vi "CRDS Server.vi"(10 "nCRD in":refnum<class "nCRD.lvclass">, 11 "DVR In":refnum<data-value>) -> (3 "nCRD out":refnum<class "nCRD.lvclass">)   [LabVIEW 2016]
uses:
  <vilib>/MSR Consulting, LLC/General Reuse/Instrument/Instrument.lvclass
  <vilib>/MSR Consulting, LLC/General Reuse/Instrument/state.ctl
  CRD/nCRD.lvclass
  <vilib>/MSR Consulting, LLC/General Reuse/Session APIs/Session Log/System Log.lvclass
  <vilib>/MSR Consulting, LLC/General Reuse/Session APIs/_Session Fwk/Session - Root.lvclass
  <vilib>/MSR Consulting, LLC/General Reuse/Session APIs/File Access/Config Data/Config Data.lvclass
  C:/Program Files (x86)/National Instruments/LabVIEW 2016/vi.lib/MSR Consulting, LLC/General Reuse/CRDS/Main/CRDS.lvclass
  C:/Program Files (x86)/National Instruments/LabVIEW 2016/vi.lib/MSR Consulting, LLC/General Reuse/Instrument/Instrument.lvclass
  C:/Program Files (x86)/National Instruments/LabVIEW 2016/vi.lib/MSR Consulting, LLC/General Reuse/Session APIs/_Session Fwk/Session - Root.lvclass
  Data/Nicholas Data.lvclass
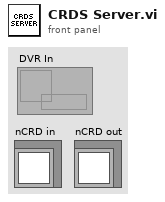
[diagram p1: front panel]
types:
  T1 = typedef "Instrument.lvclass/state.ctl" = enum8{"Configure", "Acquire", "Wait", "Quit", "Handle Error", "NOOP"}
  T2 = typedef "Session - Root.lvclass/Session Handle.ctl" = refnum<data-value>
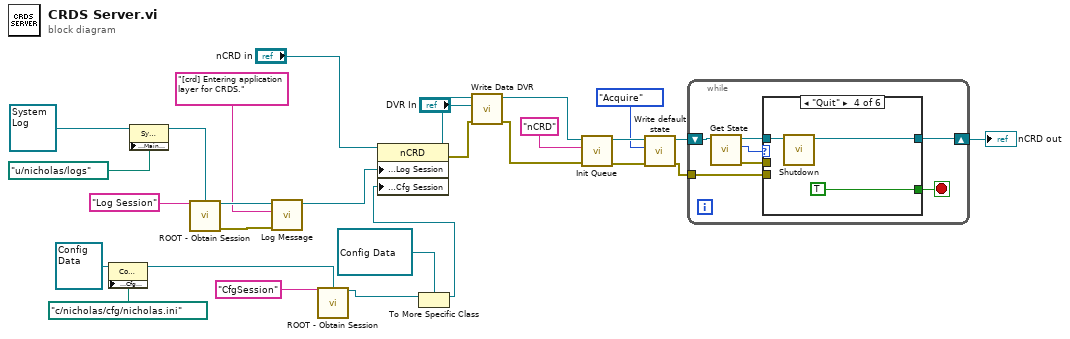
[diagram p0: block diagram]
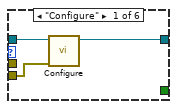
[diagram p2: hidden frame]
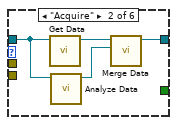
[diagram p3: hidden frame]
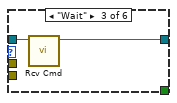
[diagram p4: hidden frame]
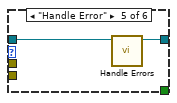
[diagram p5: hidden frame]
diagram:
  n1 = property class="Config Data"(reference=refnum<class "Config Data.lvclass"> refnum ("Config Data"), "Accessors:Cfg Path"=path "c:/nicholas/cfg/nicholas.ini" ("Cfg Path")) -> (reference out=w8:refnum<class "Config Data.lvclass">)  [unwired: 1 in, 1 out]
  n2 = property class="Sys Log"(reference=refnum<class "System Log.lvclass"> refnum ("Sys Log"), "Accessors:Main Path"=path "u:/nicholas/logs" ("Main Path")) -> (reference out=w16:refnum<class "System Log.lvclass">)  [unwired: 1 in, 1 out]
  n3 = call <vilib>:"ROOT - Obtain Session.vi"("Session Name ()"="Log Session", "OBJ - Session"=w16) -> ("Session Handle"=w13:T2, "error out"=w12:errorcluster)  [unwired: 11 in, 1 out]
  n4 = call <vilib>:"Log Message.vi"("error in"=w12, "MSG In"="[crd] Entering application layer for CRDS.", "session in"=w13) -> ("session out"=w10:T2)  [unwired: 7 in, 1 out]
  n5 = call <vilib>:"ROOT - Obtain Session.vi"("Session Name ()"="CfgSession", "OBJ - Session"=w8) -> ("Session Handle"=w3:T2)  [unwired: 11 in, 2 out]
  n6 = To More Specific Class(target class=refnum<data-value> refnum, reference=w3) -> (specific class reference=w1:refnum<data-value>)  [unwired: 1 in, 1 out]
  n7 = property class="nCRD"(reference="nCRD in", "Accessors:Log Session"=w10, "Accessors:Cfg Session"=w1) -> (reference out=w14:refnum<class "nCRD.lvclass">, error out=w5:errorcluster)  [unwired: 1 in]
  n8 = call "Write Data DVR.vi"("error in (no error)"=w5, "Data DVR"="DVR In", "nCRD in"=w14) -> ("error out"=w19:errorcluster, "nCRD out"=w28:refnum<class "nCRD.lvclass">)  [unwired: 7 in]
  n9 = call <vilib>:"Init Queue.vi"("error in"=w19, "queue_name"="nCRD", "Instrument in"=w28) -> ("error out"=w26:errorcluster, "Instrument out"=w25:refnum<class "nCRD.lvclass">)  [unwired: 7 in]
  n10 = call <vilib>:"Write default state.vi"("error in (no error)"=w26, "instr state"=state."Acquire", "Instrument in"=w25) -> ("error out"=w24:errorcluster, "Instrument out"=w23:refnum<class "nCRD.lvclass">)  [unwired: 7 in]
  n11 = while {
    shift-right: [w31] -> w20
    shift-left: w23 -> [w32]
    tunnel: w24 -> [w30]
    stop <- w34 stop-if-true
    n12 = call <vilib>:"Get State.vi"("Instrument in"=w32) -> ("error out"=w29:errorcluster, "default state"=w35:T1, "Instrument out"=w33:refnum<class "nCRD.lvclass">)  [unwired: 8 in]
    n13 = case shown="\"Quit\"" w35 {
      tunnel: [_ _ _ TRUE _ _] -> w34
      tunnel: w33 -> [w38 w42 w44 w46 w49 w50]
      tunnel: [w37 w41 w43 w45 w48 w50] -> w31
      tunnel: w30 -> [w36 _ _ _ _ _]
      tunnel: w29 -> [_ _ _ _ _ _]
      frame "Configure" {
        n14 = call-dynamic "Configure.vi"("error in"=w36, "nCRD in"=w38) -> ("nCRD out"=w37:refnum<class "nCRD.lvclass">)  [unwired: 8 in, 1 out]
      }
      frame "Acquire" {
        n15 = call-dynamic "Get Data.vi"("nCRD in"=w42) -> ("nCRD out"=w40:refnum<class "nCRD.lvclass">)  [unwired: 9 in, 1 out]
        n16 = call-dynamic "Analyze Data.vi"("nCRD in"=w42) -> ("nCRD out"=w39:refnum<class "nCRD.lvclass">)  [unwired: 9 in, 1 out]
        n17 = call-dynamic "Merge Data.vi"("Analyzed"=w39, "Acquired"=w40) -> ("CRDS out"=w41:refnum<class "nCRD.lvclass">)  [unwired: 8 in, 1 out]
      }
      frame "Wait" {
        n18 = call-dynamic "Rcv Cmd.vi"("nCRD in"=w44) -> ("nCRD out"=w43:refnum<class "nCRD.lvclass">)  [unwired: 9 in, 1 out]
      }
      frame "Quit" {
        n19 = call-dynamic "Shutdown.vi"("nCRD in"=w46) -> ("nCRD out"=w45:refnum<class "nCRD.lvclass">)  [unwired: 9 in, 1 out]
      }
      frame "Handle Error" {
        n20 = call-dynamic "Handle Errors.vi"("nCRD in"=w49) -> ("nCRD out"=w48:refnum<class "nCRD.lvclass">)  [unwired: 8 in, 2 out]
      }
      frame "NOOP", Default {
      }
    }
  }
  "nCRD out" <- w20
